vi "GetCurrentPosition.vi"(0 "VISA resource name in":refnum<visa-resource-name>, 11 "error in":errorcluster) -> (4 "VISA resource name out":refnum<visa-resource-name>, 6 "X Position":i32[](array[numeric]), 8 "Y Position":i32[](array[numeric]), 10 "Z Position":i32[](array[numeric]), 15 "error out":errorcluster)   [LabVIEW 2011]
doc: "The Basic Serial Read and Write example performs a Serial Port Read, a Serial Port Write, or a combination of these actions. The user selects the actions (read or write) on the front panel. If both are selected, the VI will write the data first, read data, and then close the VISA session that is opened to the port. This VI will wait until the specified number of bytes is received at the port or until a termination character is read.\n\nINSTRUCTIONS:\n1) Select the serial resource and configuration parameters (baud rate, data bits, parity, stop bits, flow control).\n2) Select the operations to be performed. \n3) Connect the serial port to your device. If no device is available, perform a loopback test by doing one of the following. Short pins 2 and 3 on a RS-232 cable or short pin 4 to pin 8 and pin 5 to pin 9 on a RS-485/422 cable. \n4) Run the VI to see the data read. (The \"read string\" will match the \"string to write\" if a loopback test was performed.)\n\nNote: The parameters set for the serial port must match the parameters of the connected instrument or device. In this example, the bytes to read parameter specifies the number of bytes that the serial port reads. If there were more bytes at the port than the number specified in bytes to read, those bytes would not be read. Also, if you specify to read more bytes than the number of bytes actually read, you might receive a timeout error message.\n\nOn the block diagram, the Configure Serial Port VI sets the configuration parameters. The front panel displays the controls used to configure the basic parameters, such as baud rate, data bits, and parity. Constants configure the other parameters the user probably does not need set. After the VISA Configure Serial Port VI opens the VISA session and configures the port, the VI passes the VISA resource name to other VIs that perform operations on that VISA resource. The VISA Write function sends a command to the serial device and the VISA Read function returns data based on the command. The VISA Close function then closes the reference to the serial device. It is important to close the reference; otherwise communication through with that port through protocols other than VISA might not be possible."
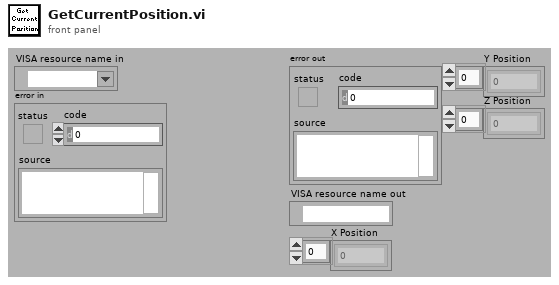
[diagram p1: front panel]
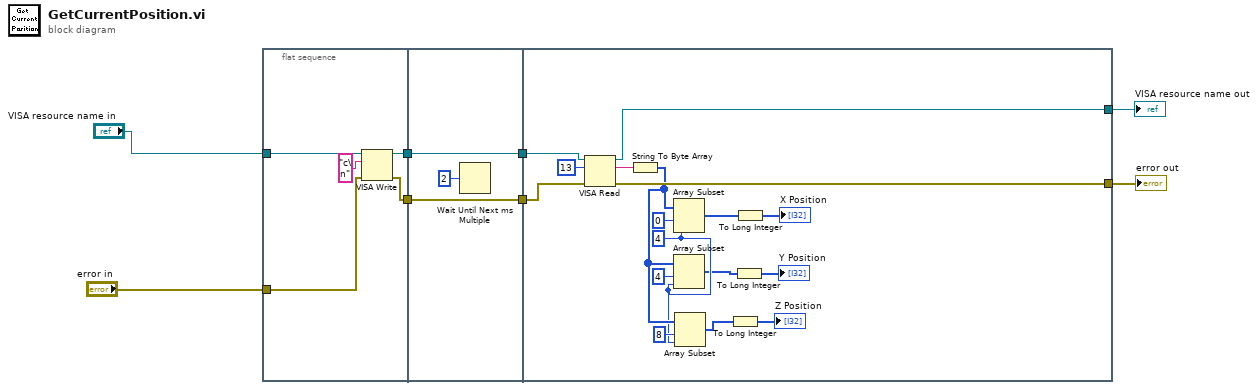
[diagram p0: block diagram]
diagram:
  n1 = flat-sequence {
    tunnel: "VISA resource name in" -> [w11]
    tunnel: "error in" -> [w12]
    tunnel: [w10] -> w6
    tunnel: [w9] -> w3
    tunnel: w6 -> [w15]
    tunnel: [w15] -> w5
    tunnel: w3 -> [w14]
    tunnel: [w14] -> w2
    tunnel: w5 -> [w33]
    tunnel: [w31] -> w4
    tunnel: w2 -> [w30]
    tunnel: [w29] -> w1
    frame #0 {
      n2 = VISA Write(VISA resource name=w11, write buffer="c\n", error in (no error)=w12) -> (VISA resource name out=w10:refnum<visa-resource-name>, error out=w9:errorcluster)  [unwired: 1 out]
    }
    frame #1 {
      n3 = Wait Until Next ms Multiple(millisecond multiple=u32 2) -> ()  [unwired: 1 out]
    }
    frame #2 {
      w22 = 4 ("length")
      n4 = VISA Read(VISA resource name=w33, byte count=u32 13, error in (no error)=w30) -> (VISA resource name out=w29:refnum<visa-resource-name>, read buffer=w28:string, error out=w31:errorcluster)  [unwired: 1 out]
      n5 = String To Byte Array(string=w28) -> (unsigned byte array=w25:u8[])
      n6 = Array Subset(array=w25, index=0, length=w22) -> (w26:u8[])
      n7 = Array Subset(array=w25, index=4, length=w22) -> (w20:u8[])
      n8 = Array Subset(array=w25, index=8, length=w22) -> (w21:u8[])
      n9 = To Long Integer(number=w21) -> (32bit integer=→"Z Position":i32[])
      n10 = To Long Integer(number=w20) -> (32bit integer=→"Y Position":i32[])
      n11 = To Long Integer(number=w26) -> (32bit integer=→"X Position":i32[])
    }
  }
  "error out" <- w4
  "VISA resource name out" <- w1
